vi "2D Gaussian fitting model.vi"(3 "output control":T1 caption="输出控制", 4 "data":variant caption="数据", 5 "X":dbl[](array[numeric]), 6 "a":dbl[](array[numeric])) -> (0 "error out":errorcluster caption="错误输出", 1 "f'(X,a)":dbl[][](array[numeric]), 2 "f(X,a)":dbl[](array[numeric]))   [LabVIEW 2015]
doc: "This template is the starting point for creating a model function to be passed to the Nonlinear Curve Fit.vi."
uses:
  <vilib>/gmath/NumericalOptimization/LM_output select.ctl
  <vilib>/gmath/NI_Gmath.lvlib
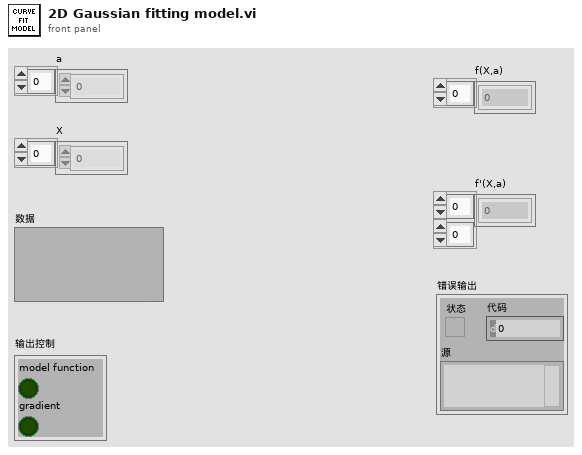
[diagram p1: front panel]
types:
  T1 = typedef "NI_Gmath.lvlib/LM_output select.ctl" = cluster{"model function":bool, "gradient":bool}
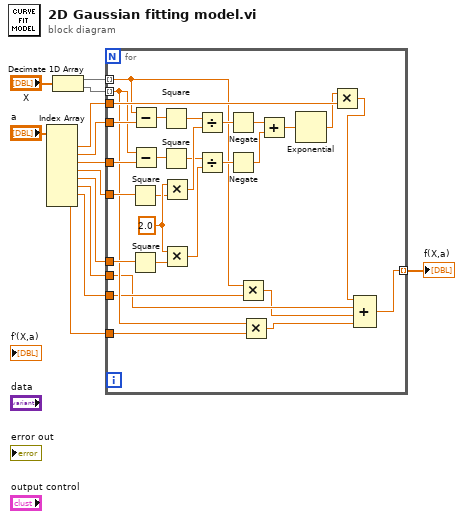
[diagram p0: block diagram]
diagram:
  n1 = Index Array(array="a") -> (element #1=w12:dbl, element #2=w11:dbl, element #3=w10:dbl, element #4=w9:dbl, element #5=w8:dbl, element #6=w7:dbl, element #7=w2:dbl, element #8=w1:dbl)  [unwired: 8 in]
  n2 = Decimate 1D Array("X") -> (w5:dbl[], w4:dbl[])
  n3 = for {
    tunnel: w12 -> [w24]
    tunnel: w11 -> [w41]
    tunnel: w10 -> [w42]
    tunnel: w9 -> [w36]
    tunnel: w8 -> [w37]
    tunnel: w7 -> [w17]
    tunnel: w5 -> [w22] mode=indexing
    tunnel: w4 -> [w21] mode=indexing
    tunnel: [w14] -> w3 mode=indexing
    tunnel: w2 -> [w20]
    tunnel: w1 -> [w19]
    w38 = 2.0 ("x")
    n4 = Square(x=w36) -> (x^2=w35:dbl)
    n5 = Square(x=w37) -> (x^2=w34:dbl)
    n6 = Subtract(x=w22, y=w41) -> (x-y=w40:dbl)
    n7 = Subtract(x=w21, y=w42) -> (x-y=w39:dbl)
    n8 = Square(x=w40) -> (x^2=w33:dbl)
    n9 = Square(x=w39) -> (x^2=w31:dbl)
    n10 = Multiply(x=w38, y=w35) -> (x*y=w32:dbl)
    n11 = Multiply(x=w38, y=w34) -> (x*y=w30:dbl)
    n12 = Divide(x=w33, y=w32) -> (x/y=w29:dbl)
    n13 = Divide(x=w31, y=w30) -> (x/y=w28:dbl)
    n14 = Negate(x=w29) -> (-x=w27:dbl)
    n15 = Negate(x=w28) -> (-x=w26:dbl)
    n16 = Multiply(x=w22, y=w20) -> (x*y=w16:dbl)
    n17 = Multiply(x=w21, y=w19) -> (x*y=w15:dbl)
    n18 = Add(x=w27, y=w26) -> (x+y=w25:dbl)
    n19 = Exponential(1:w25) -> (0:w23:dbl)
    n20 = Multiply(x=w23, y=w24) -> (x*y=w18:dbl)
    n21 = Compound Arithmetic op=ADD(w18, w17, w16, w15) -> (w14:dbl)
  }
  "f(X,a)" <- w3
